vi "sequence simple.vi"() -> ()   [LabVIEW 2015]
uses:
  result/result.lvclass
  result/result.lvclass/result.ctl
  result/get data.vi
  result/get error.vi
  result/get subresults.vi
  result/get owning task.vi
  task/task.lvclass
  dispatcher/thread pool.lvclass
  standard reporters/event reporter/event reporter.lvclass
  standard tasks/sequence task/sequence task.lvclass
  standard action/wait action/wait action.lvclass
panel:
  out "x = y?":bool[](array[boolean])
  out "error":errorcluster
  out "data":variant
  out "accessors:subresults":refnum<class "result.lvclass">[][](array[class])
  out "Array 2":errorcluster[](array[cluster])
  out "Array":variant[](array[variant])
  out "Time":u32
  out "result":refnum<class "result.lvclass">
  out "error out":errorcluster
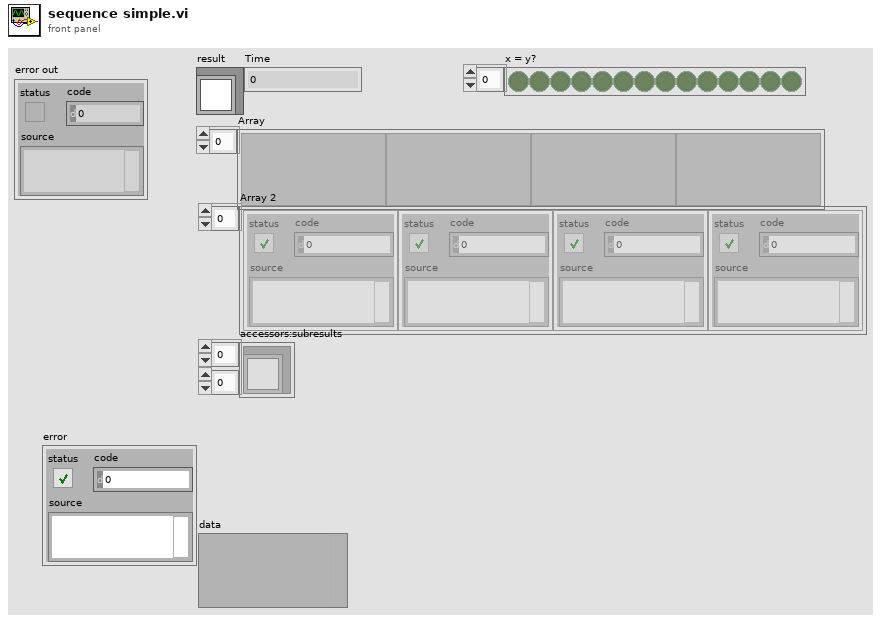
[diagram p1: front panel]
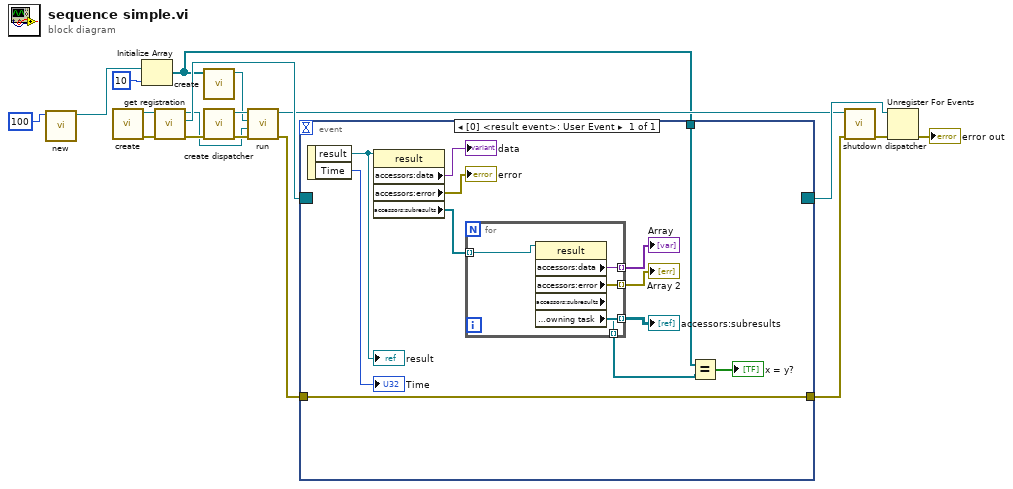
[diagram p0: block diagram]
diagram:
  n1 = call "new.vi"("timer"=100) -> ("wait action out"=w4:refnum<class "wait action.lvclass">)  [unwired: 10 in]
  n2 = call "create.vi"() -> ("error out"=w15:errorcluster, "event reporter out"=w16:refnum<class "event reporter.lvclass">)  [unwired: 10 in]
  n3 = Initialize Array(w4, 10 ("dimension size")) -> (w1:refnum<class "wait action.lvclass">[])
  n4 = call "get registration.vi"("error in"=w15, "event reporter in"=w16) -> ("error out"=w14:errorcluster, "result registration"=w13:refnum<event-registration>, "event reporter out"=w2:refnum<class "event reporter.lvclass">)  [unwired: 7 in]
  n5 = call "create.vi"("tasks"=w1) -> ("sequence task out"=w5:refnum<class "sequence task.lvclass">)  [unwired: 10 in]
  n6 = call "create dispatcher.vi"("error in"=w14) -> ("error out"=w17:errorcluster, "dispatcher"=w18:refnum<class "thread pool.lvclass">)  [unwired: 9 in]
  n7 = call "run.vi"("error in"=w17, "results reporter"=w2, "task"=w5, "thread pool in"=w18) -> ("error out"=w7:errorcluster, "thread pool out"=w11:refnum<class "thread pool.lvclass">)  [unwired: 6 in]
  n8 = event shown="[0] <result event>: User Event" {
    selector: w13 -> [_]
    dyn-events: [_] -> w12
    timeout: _ -> [_]
    tunnel: [w29] -> w8
    tunnel: w7 -> [w29]
    tunnel: w1 -> [w21]
    event User Event {
      n9 = event-data() -> ("result"=w28:refnum<class "result.lvclass">, "Time"=→"Time":u32)  [unwired: 1 in]
      "result" <- w28
      n10 = property class="result"(reference=w28) -> ("accessors:data"=→"data":variant, "accessors:error"=→"error":errorcluster, "accessors:subresults"=w27:refnum<class "result.lvclass">[])  [unwired: 1 in, 2 out]
      n11 = for {
        tunnel: w27 -> [w35] mode=indexing
        tunnel: [w34] -> w26 mode=indexing
        tunnel: [w33] -> w25 mode=indexing
        tunnel: [w32] -> w24 mode=indexing
        tunnel: [w31] -> w20 mode=indexing
        n12 = property class="result"(reference=w35) -> ("accessors:data"=w34:variant, "accessors:error"=w33:errorcluster, "accessors:subresults"=w32:refnum<class "result.lvclass">[], "accessors:owning task"=w31:refnum<class "task.lvclass">)  [unwired: 1 in, 2 out]
      }
      "Array" <- w26
      "Array 2" <- w25
      "accessors:subresults" <- w24
      n13 = Equal?(x=w21, y=w20) -> (x = y?=→"x = y?":bool[])
    }
  }
  n14 = call "shutdown dispatcher.vi"("error in"=w8, "thread pool"=w11) -> ("error out"=w10:errorcluster)  [unwired: 9 in]
  n15 = Unregister For Events(event registration refnum=w12, error in=w10) -> (error out=→"error out":errorcluster)
